vi "CNT_VI_Test.vi"() -> ()   [LabVIEW 2020]
panel:
  out "AtoD":i16(knob) scale=-8192.0..8191.0
  in  "stop":bool
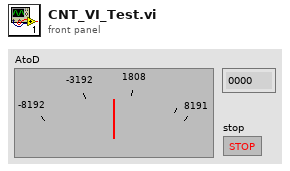
[diagram p1: front panel]
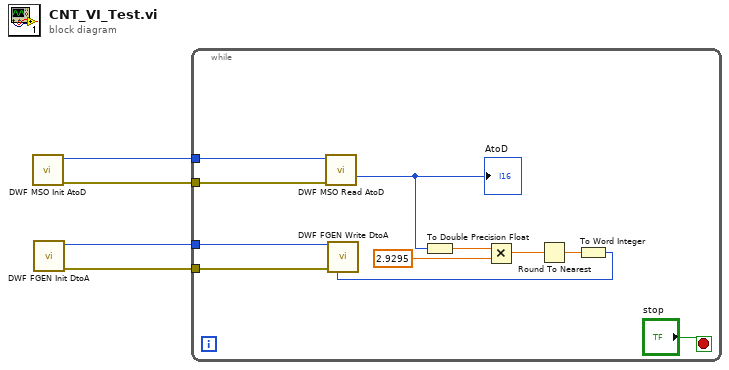
[diagram p0: block diagram]
diagram:
  n1 = call "DWF MSO Init AtoD.vi"() -> ("Error Out"=w3:errorcluster, "Instrument Handle Out"=w4:u32)  [unwired: 10 in]
  n2 = call "DWF FGEN Init DtoA.vi"() -> ("Error Out"=w1:errorcluster, "Instrument Handle Out"=w2:u32)  [unwired: 10 in]
  n3 = while {
    tunnel: w4 -> [w14]
    tunnel: w3 -> [w13]
    tunnel: w2 -> [w12]
    tunnel: w1 -> [w11]
    stop <- "stop" stop-if-true
    n4 = call "DWF MSO Read AtoD.vi"("Instrument Handle In AtoD"=w14, "Error In"=w13) -> ("AtoD"=w10:i16)  [unwired: 12 in, 1 out]
    "AtoD" <- w10
    n5 = To Double Precision Float(number=w10) -> (double precision float=w9:dbl)
    n6 = Multiply(x=w9, y=2.9295) -> (x*y=w7:dbl)
    n7 = Round To Nearest(number=w7) -> (nearest integer value=w6:dbl)
    n8 = To Word Integer(number=w6) -> (16bit integer=w5:i16)
    n9 = call "DWF FGEN Write DtoA.vi"("Instrument Handle In"=w12, "Error In"=w11, "Raw Data"=w5) -> ()  [unwired: 11 in, 2 out]
  }
